vi "Vehicle Position Simulation.vi"() -> ()   [LabVIEW 2017]
panel:
  in  "Vehicle Position Simulation":i8(slide) min=0 max=4 step=1 scale=0.0..4.0
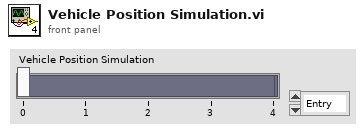
[diagram p1: front panel]
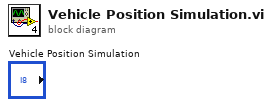
[diagram p0: block diagram]
diagram:
